vi "AtlasHTTP.vi"(0 "error in (no error)":errorcluster, 2 "Laser":u16(ring) items=["Minerva", "Neptune", "Jupiter"], 3 "Command":u16(ring)=2 items=["Login", "Logout", "get_laser_names", "Ping", "Unlock", "Lock171", "Lock174", "Connect", "Disconnect"]) -> (6 "error out":errorcluster, 8 "body":string)   [LabVIEW 2019]
uses:
  <vilib>/httpClient/LabVIEWHTTPClient.lvlib
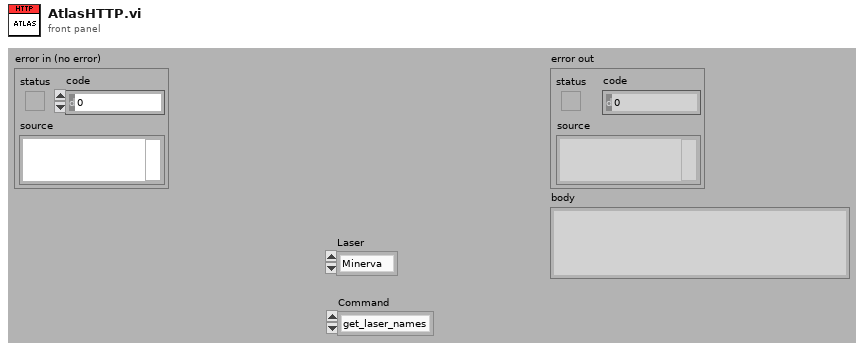
[diagram p1: front panel]
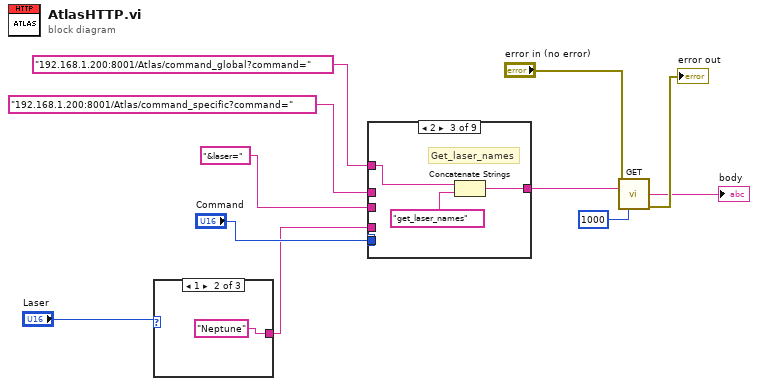
[diagram p0: block diagram]
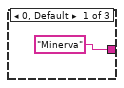
[diagram p2: hidden frame]
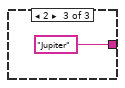
[diagram p3: hidden frame]
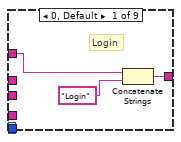
[diagram p4: hidden frame]
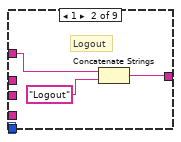
[diagram p5: hidden frame]
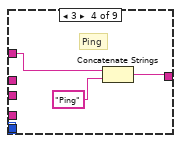
[diagram p6: hidden frame]
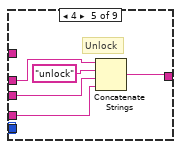
[diagram p7: hidden frame]
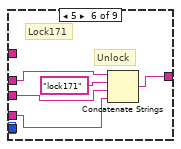
[diagram p8: hidden frame]
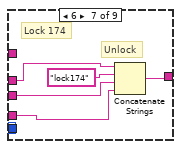
[diagram p9: hidden frame]
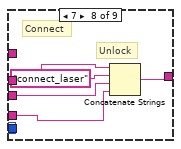
[diagram p10: hidden frame]
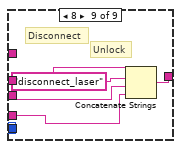
[diagram p11: hidden frame]
diagram:
  n1 = case shown="1" "Laser" {
    tunnel: ["Minerva" "Neptune" "Jupiter"] -> w5
    frame 0, Default {
    }
    frame 1 {
    }
    frame 2 {
    }
  }
  n2 = case shown="2" "Command" {
    tunnel: "Command" -> [_ _ _ _ _ _ _ _ _]
    tunnel: [w15 w19 w23 w24 w27 w32 w40 w45 w50] -> w11
    tunnel: "192.168.1.200:8001/Atlas/command_global?command=" -> [w16 w18 w22 w25 _ _ _ _ _]
    tunnel: "192.168.1.200:8001/Atlas/command_specific?command=" -> [_ _ _ _ w30 w35 w37 w44 w49]
    tunnel: "&laser=" -> [_ _ _ _ w29 w34 w38 w42 w48]
    tunnel: w5 -> [_ _ _ _ w28 w33 w39 w43 w47]
    frame 0, Default {
      # "Login"
      n3 = Concatenate Strings(w16, "Login" ("string")) -> (w15:string)
    }
    frame 1 {
      # "Logout"
      n4 = Concatenate Strings(w18, "Logout" ("string")) -> (w19:string)
    }
    frame 2 {
      # "Get_laser_names"
      n5 = Concatenate Strings(w22, "get_laser_names" ("string")) -> (w23:string)
    }
    frame 3 {
      # "Ping"
      n6 = Concatenate Strings(w25, "Ping" ("string")) -> (w24:string)
    }
    frame 4 {
      # "Unlock"
      n7 = Concatenate Strings(w30, "unlock" ("string"), w29, w28) -> (w27:string)
    }
    frame 5 {
      # "Unlock"
      # "Lock171"
      n8 = Concatenate Strings(w35, "lock171" ("string"), w34, w33) -> (w32:string)
    }
    frame 6 {
      # "Unlock"
      # "Lock 174"
      n9 = Concatenate Strings(w37, "lock174" ("string"), w38, w39) -> (w40:string)
    }
    frame 7 {
      # "Unlock"
      # "Connect"
      n10 = Concatenate Strings(w44, "connect_laser" ("string"), w42, w43) -> (w45:string)
    }
    frame 8 {
      # "Unlock"
      # "Disconnect"
      n11 = Concatenate Strings(w49, "disconnect_laser" ("string"), w48, w47) -> (w50:string)
    }
  }
  n12 = call <vilib>:"GET.vi"("url"=w11, "error in (no error)"="error in (no error)", "timeout (10000)"=1000) -> ("body"=→"body":string, "error out"=→"error out":errorcluster)  [unwired: 9 in, 2 out]
